vi "creadorenomstring.vi"(10 "cadena":string[](array[string])) -> (1 "adquisicion":string[](array[string]), 2 "control":string[](array[string]))   [LabVIEW 2016]
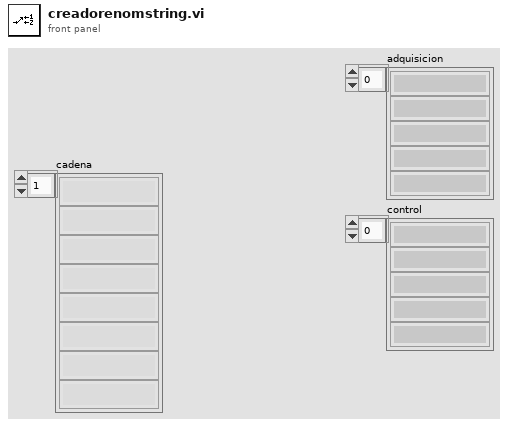
[diagram p1: front panel]
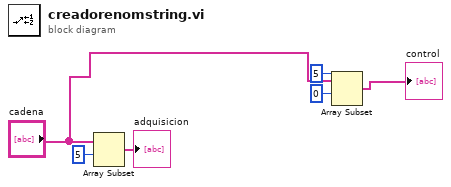
[diagram p0: block diagram]
diagram:
  n1 = Array Subset(array="cadena", index=5) -> (→"adquisicion":string[])  [unwired: 1 in]
  n2 = Array Subset(array="cadena", index=0, length=5) -> (→"control":string[])
